vi "Array to Spectrum (N Ch).vi"(8 "channel names":string[](array[string]), 9 "f0":dbl, 10 "df":dbl, 11 "array":dbl[](array[numeric])) -> (3 "spectra":cluster{"x0":dbl, "dx":dbl, "magnitude":dbl[]}[](array[cluster]))   [LabVIEW 2021]
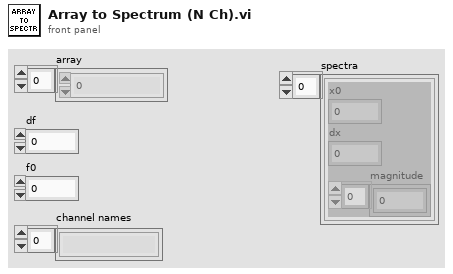
[diagram p1: front panel]
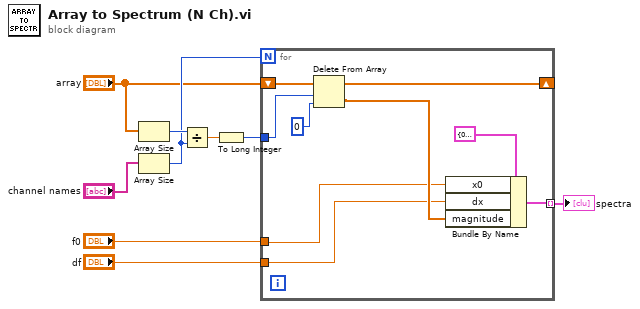
[diagram p0: block diagram]
diagram:
  n1 = Array Size(array="array") -> (size(s)=w9:i32)
  n2 = Array Size(array="channel names") -> (size(s)=w8:i32)
  n3 = Divide(x=w9, y=w8) -> (x/y=w6:dbl)
  n4 = To Long Integer(number=w6) -> (32bit integer=w5:i32)
  n5 = for {
    N: w8 -> [_]
    shift-right: [w17] -> _
    shift-left: "array" -> [w18]
    tunnel: w5 -> [w15]
    tunnel: "df" -> [w10]
    tunnel: [w14] -> w1 mode=indexing
    tunnel: "f0" -> [w11]
    n6 = Delete From Array(array=w18, length=w15, index=0) -> (deleted portion=w12:dbl[], array with subset deleted=w17:dbl[])
    n7 = Bundle By Name(cluster=cluster{"x0":dbl, "dx":dbl, "magnitude":dbl[]} {"x0"=0.0, "dx"=0.0, "magnitude"=[]} ("converted spectrum"), "x0"=w11, "dx"=w10, "magnitude"=w12) -> (w14:cluster{"x0":dbl, "dx":dbl, "magnitude":dbl[]})
  }
  "spectra" <- w1
